vi "dataset.get.vi"(8 "error in":errorcluster, 10 "Datascope Name":string, 11 "asset in":refnum<class "asset.lvclass">) -> (0 "error out":errorcluster, 2 "dataset":refnum<class "dataset.lvclass">, 3 "asset out":refnum<class "asset.lvclass">)   [LabVIEW 2020, in "asset.lvclass"]
uses:
  asset.lvclass
  Nominal Client/datasources/dataset/dataset.lvclass
  asset.lvclass/asset.ctl
  Nominal Client/datasources/dataset/dataset.lvclass/dataset.ctl
  Nominal Client/datasources/dataset/rid.get.vi
  Nominal Client/Nominal Client.lvclass
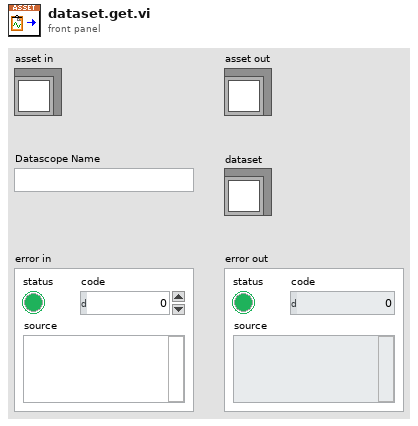
[diagram p1: front panel]
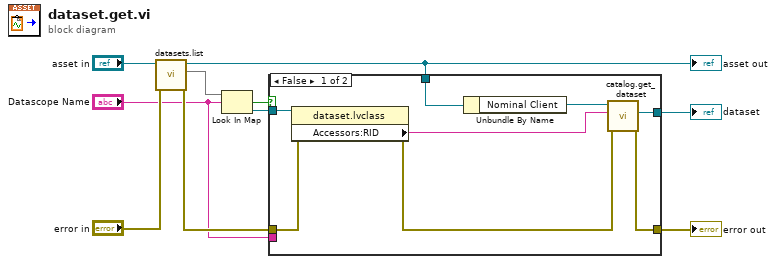
[diagram p0: block diagram]
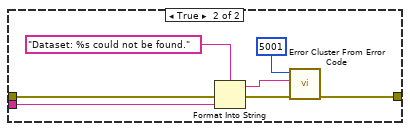
[diagram p2: hidden frame]
diagram:
  n1 = call "datasets.list.vi"("error in"="error in", "asset in"="asset in") -> ("error out"=w7:errorcluster, "datasets"=w9:map{string, refnum<class "dataset.lvclass">}, "asset out"=w3:refnum<class "asset.lvclass">)  [unwired: 7 in]
  "asset out" <- w3
  n2 = Look In Map(map=w9, key="Datascope Name") -> (key not found?=w6:bool, value=w4:refnum<class "dataset.lvclass">)  [unwired: 1 in]
  n3 = case shown="False" w6 {
    tunnel: "Datascope Name" -> [_ w23]
    tunnel: [w13 w20] -> w1
    tunnel: w7 -> [w11 w19]
    tunnel: w4 -> [w17 _]
    tunnel: w3 -> [w16 _]
    tunnel: [w15 _] -> w2
    frame False {
      n4 = property class="dataset.lvclass"(reference=w17, error in=w11) -> (error out=w12:errorcluster, "Accessors:RID"=w14:string)  [unwired: 1 out]
      n5 = Unbundle By Name(w16) -> ("Nominal Client"=w18:refnum<class "Nominal Client.lvclass">)
      n6 = call "catalog.get_dataset.vi"("error in"=w12, "Dataset UUID"=w14, "Nominal Client in"=w18) -> ("error out"=w13:errorcluster, "Dataset"=w15:refnum<class "dataset.lvclass">)  [unwired: 6 in, 1 out]
    }
    frame True {
      n7 = Format Into String(format string="Dataset: %s could not be found.", error in=w19, w23) -> (resulting string=w22:string, error out=w21:errorcluster)  [unwired: 1 in]
      n8 = call <vilib>:"Error Cluster From Error Code.vi"("error in (no error)"=w21, "error message (\"\")"=w22, "error code (0)"=5001) -> ("error out"=w20:errorcluster)  [unwired: 6 in]
    }
  }
  "error out" <- w1
  "dataset" <- w2
